vi "CMD_POW.vi"(6 "Gantry in":refnum<class "Gantry.lvclass">, 8 "error in (no error)":errorcluster, 10 "Arguments":string[](array[string]), 11 "gScript Interpreter in":refnum<class "gScript Interpreter.lvclass">) -> (0 "error out":errorcluster, 3 "gScript Interpreter out":refnum<class "gScript Interpreter.lvclass">, 4 "Gantry out":refnum<class "Gantry.lvclass">)   [LabVIEW 2023, in "gScript Interpreter.lvclass"]
uses:
  gScript Interpreter.lvclass
  Shared Components/Gantry Class/Gantry.lvclass
  Type Definitions/Memory Cell.ctl
  Type Definitions/Memory Cell Type Enum.ctl
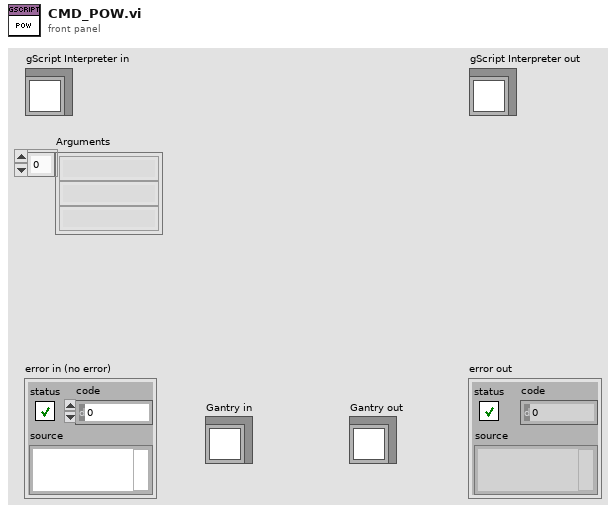
[diagram p1: front panel]
types:
  T1 = typedef "Memory Cell Type Enum.ctl" = enum16{"integer", "float", "vector", "rotation"}
  T2 = typedef "Memory Cell.ctl" = cluster{"type":T1, "x":dbl, "y":dbl, "z":dbl, "w":dbl}
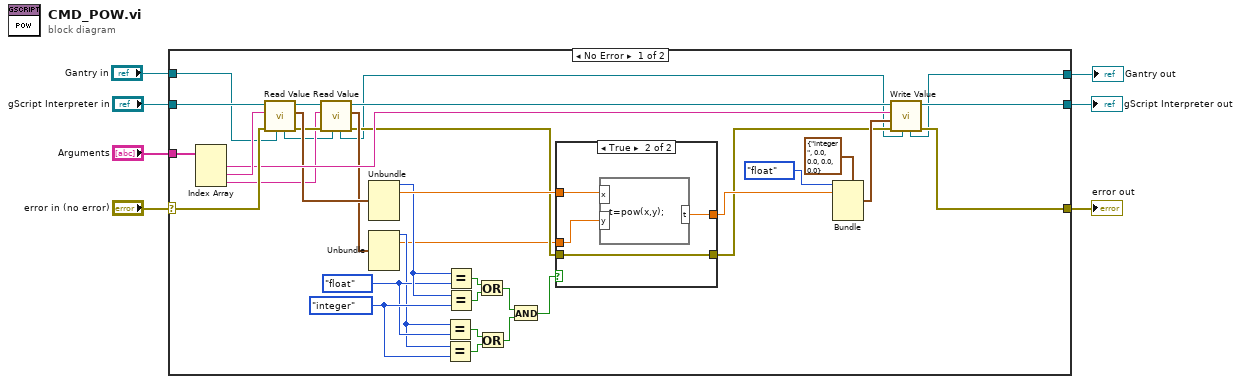
[diagram p0: block diagram]
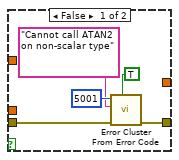
[diagram p2: hidden frame]
diagram:
  n1 = case shown="No Error" "error in (no error)" {
    selector: "error in (no error)" -> [w41 w55]
    tunnel: [w34 w55] -> w6
    tunnel: [w35 w54] -> w4
    tunnel: "gScript Interpreter in" -> [w42 w54]
    tunnel: "Arguments" -> [w43 _]
    tunnel: "Gantry in" -> [w11 w53]
    tunnel: [w8 w53] -> w1
    frame No Error {
      w22 = Memory_Cell_Type_Enum."integer" ("type")
      w21 = Memory_Cell_Type_Enum."float" ("type")
      n2 = Index Array(array=w43) -> (element #1=w39:string, element #2=w40:string, element #3=w27:string)  [unwired: 3 in]
      n3 = call-dynamic "Read Value.vi"("Gantry in"=w11, "error in (no error)"=w41, "String in"=w40, "gScript Interpreter in"=w42) -> ("error out"=w28:errorcluster, "Memory Cell"=w38:T2, "gScript Interpreter out"=w29:refnum<class "gScript Interpreter.lvclass">, "Gantry out"=w10:refnum<class "Gantry.lvclass">)  [unwired: 4 in]
      n4 = call-dynamic "Read Value.vi"("Gantry in"=w10, "error in (no error)"=w28, "String in"=w27, "gScript Interpreter in"=w29) -> ("error out"=w24:errorcluster, "Memory Cell"=w26:T2, "gScript Interpreter out"=w25:refnum<class "gScript Interpreter.lvclass">, "Gantry out"=w9:refnum<class "Gantry.lvclass">)  [unwired: 4 in]
      n5 = Unbundle(w38) -> ("type"=w23:T1, "x"=w33:dbl)  [unwired: 3 out]
      n6 = Unbundle(w26) -> ("type"=w20:T1, "x"=w12:dbl)  [unwired: 3 out]
      n7 = Equal?(x=w20, y=w21) -> (x = y?=w17:bool)
      n8 = Equal?(x=w20, y=w22) -> (x = y?=w16:bool)
      n9 = Equal?(x=w23, y=w21) -> (x = y?=w18:bool)
      n10 = Equal?(x=w23, y=w22) -> (x = y?=w19:bool)
      n11 = Or(x=w18, y=w19) -> (x .or. y?=w15:bool)
      n12 = Or(x=w17, y=w16) -> (x .or. y?=w14:bool)
      n13 = And(x=w15, y=w14) -> (x .and. y?=w13:bool)
      n14 = case shown="True" w13 {
        tunnel: w33 -> [_ w51]
        tunnel: [_ w49] -> w32
        tunnel: w24 -> [w44 w52]
        tunnel: [w48 w52] -> w30
        tunnel: w12 -> [_ w50]
        frame False {
          n15 = call <vilib>:"Error Cluster From Error Code.vi"("show call chain? (False)"=TRUE, "error in (no error)"=w44, "error message (\"\")"="Cannot call ATAN2 on non-scalar type" ("error message (\"\")"), "error code (0)"=5001) -> ("error out"=w48:errorcluster)  [unwired: 5 in]
        }
        frame True {
          n16 = formula code="t=pow(x,y);"("x"=w51, "y"=w50) -> ("t"=w49:dbl)
        }
      }
      n17 = Bundle(cluster=T2 {"type"=enum."integer", "x"=0.0, "y"=0.0, "z"=0.0, "w"=0.0} ("Memory Cell"), "type"=Memory_Cell_Type_Enum."float", "x"=w32) -> (w36:T2)  [unwired: 3 in]
      n18 = call-dynamic "Write Value.vi"("Gantry in"=w9, "error in (no error)"=w30, "Value"=w36, "Address"=w39, "gScript Interpreter in"=w25) -> ("error out"=w34:errorcluster, "gScript Interpreter out"=w35:refnum<class "gScript Interpreter.lvclass">, "Gantry out"=w8:refnum<class "Gantry.lvclass">)  [unwired: 4 in]
    }
    frame Error {
    }
  }
  "error out" <- w6
  "gScript Interpreter out" <- w4
  "Gantry out" <- w1
